vi "getReconstructionDescriptor.vi"(8 "error in (no error)":errorcluster, 11 "VGS_Project in":refnum<class "VGS_Project.lvclass">) -> (0 "error out":errorcluster, 2 "ReconstructionDescriptor":refnum<k24>, 3 "VGS_Project out":refnum<class "VGS_Project.lvclass">)   [LabVIEW 2022 SP3, in "LV_VGS.lvlib" / "VGS_Project.lvclass"]
uses:
  VGS_Project.lvclass
  C:/Users/Andrey/Desktop/hajo/LV_VGS/vgs_project.dll
  vgs_project.dll
  VGS_Project.lvclass/VGS_Project.ctl
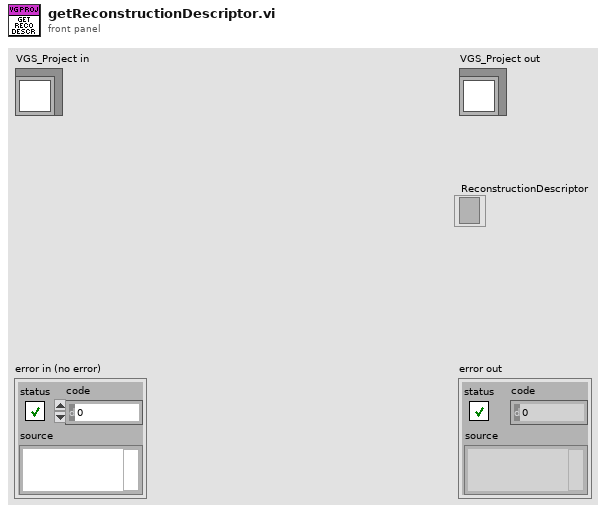
[diagram p1: front panel]
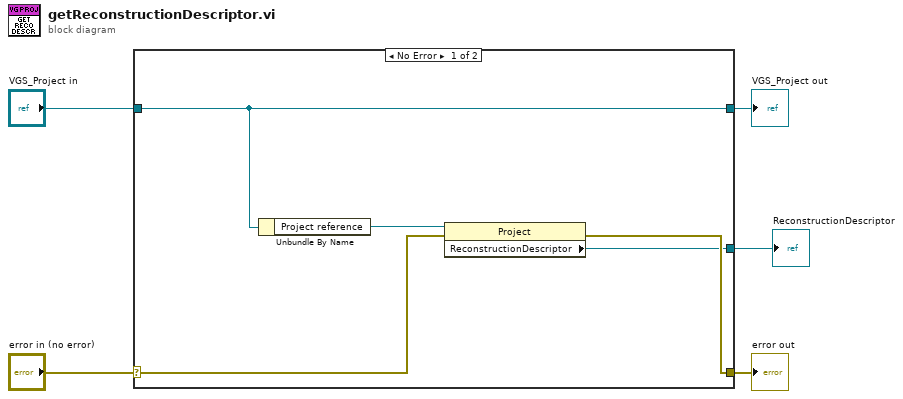
[diagram p0: block diagram]
diagram:
  n1 = case shown="No Error" "error in (no error)" {
    selector: "error in (no error)" -> [w8 w12]
    tunnel: [w7 w12] -> w4
    tunnel: [w10 w11] -> w2
    tunnel: "VGS_Project in" -> [w10 w11]
    tunnel: [w6 _] -> w1
    frame No Error {
      n2 = Unbundle By Name(w10) -> ("Project reference"=w9:refnum<k24>)
      n3 = property class="Project"(reference=w9, error in=w8) -> (error out=w7:errorcluster, "ReconstructionDescriptor"=w6:refnum<k24>)  [unwired: 1 out]
    }
    frame Error {
    }
  }
  "error out" <- w4
  "VGS_Project out" <- w2
  "ReconstructionDescriptor" <- w1
